vi "Arreglo_Cluster.vi"() -> ()   [LabVIEW 2016]
panel:
  in  "Array 2":T1(array[cluster])
  in  "Cluster":cluster{"Array":dbl[][], "Array 2":bool[][]}
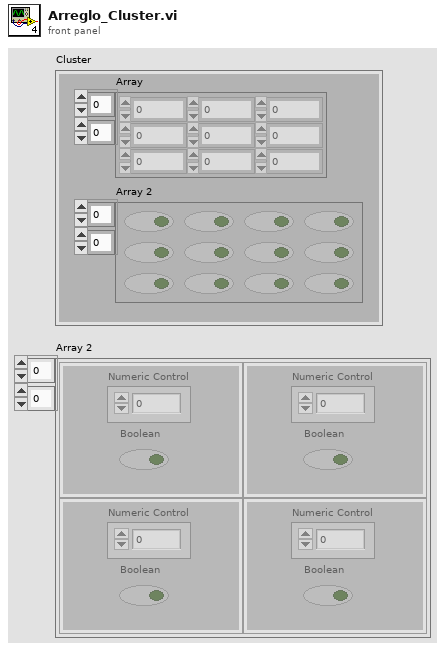
[diagram p1: front panel]
types:
  T1 = cluster{"Numeric Control":dbl, "Boolean":bool}[][]
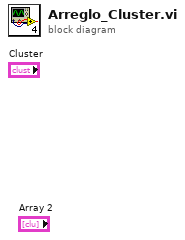
[diagram p0: block diagram]
diagram:
